vi "Destroy Connection Factory.vi"(8 "error in (no error)":errorcluster, 11 "TCP Server in":refnum<class "TCP Server.lvclass">) -> (0 "error out":errorcluster)   [LabVIEW 2019, in "TCP Interface.lvlib" / "TCP Server.lvclass"]
uses:
  <vilib>/gpm_packages/@cs/Network-Sink/Source/TCP Interface/TCP Server/TCP Server.lvclass
  <vilib>/gpm_packages/@cs/Network-Sink/Source/TCP Interface/TCP Server/TCP Server.lvclass/TCP Server.ctl
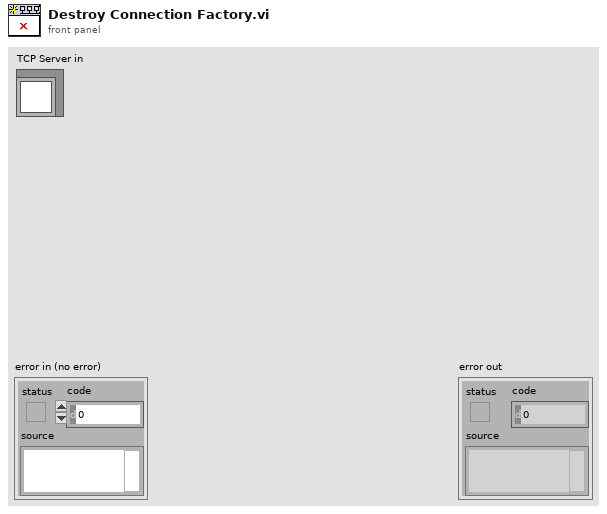
[diagram p1: front panel]
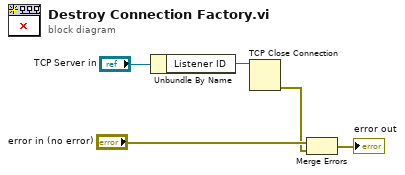
[diagram p0: block diagram]
diagram:
  n1 = Unbundle By Name("TCP Server in") -> ("Listener ID"=w3:refnum<k5>)
  n2 = TCP Close Connection(connection ID=w3) -> (error out=w1:errorcluster)  [unwired: 2 in, 1 out]
  n3 = Merge Errors("error in (no error)", w1) -> (→"error out":errorcluster)
